vi "Add RPC Memeber VIs.vi"(8 "error in":errorcluster, 9 "Member VI Template Path":path=path "C:/dev/github/codegen/grpc-labview/labview source/Client Server Support New/gRPC Scripting Tools/Class API/MemberTemplate.vi", 10 "LVClassLibrary in":refnum<vi>, 11 "RPC Method Parameters":T1[](array[typedef])) -> (0 "error out":errorcluster, 2 "dynamic member VIs":refnum<vi>[](array[refnum]), 3 "LVClassLibrary out":refnum<vi>)   [LabVIEW 2019, in "gRPC Template Creation Utility.lvlib"]
uses:
  gRPC Template Creation Utility.lvlib
  TypeDefs/RPC Method Parameters.ctl
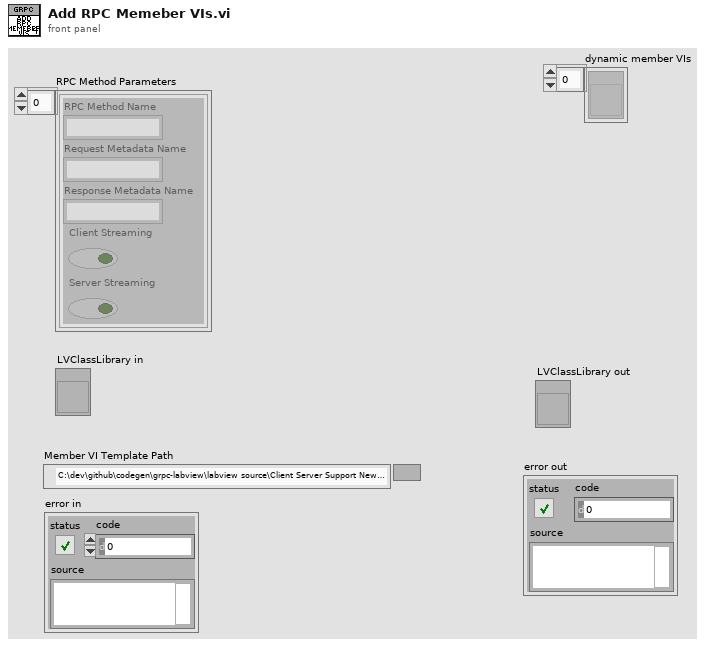
[diagram p1: front panel]
types:
  T1 = typedef "gRPC Template Creation Utility.lvlib/RPC Method Parameters.ctl" = cluster{"RPC Method Name":string, "Request Metadata Name":string, "Response Metadata Name":string, "Client Streaming":bool, "Server Streaming":bool}
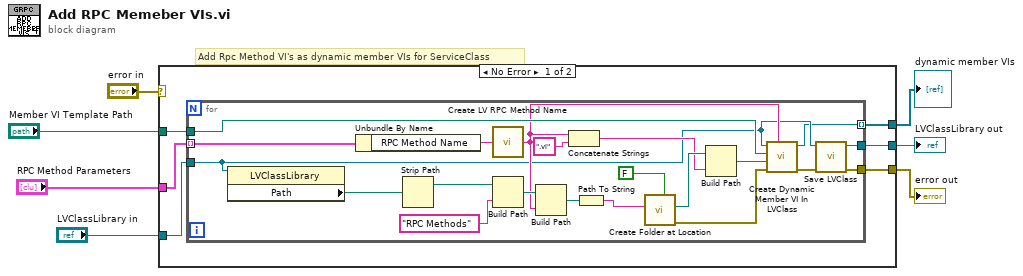
[diagram p0: block diagram]
diagram:
  # "Add Rpc Method VI's as dynamic member VIs for ServiceClass"
  n1 = case shown="No Error" "error in" {
    selector: "error in" -> [_ w36]
    tunnel: "RPC Method Parameters" -> [w13 _]
    tunnel: "LVClassLibrary in" -> [w12 w35]
    tunnel: [w11 w35] -> w4
    tunnel: "Member VI Template Path" -> [w10 _]
    tunnel: [w9 w36] -> w2
    tunnel: [w8 _] -> w1
    frame No Error {
      n2 = for {
        tunnel: w13 -> [w34] mode=indexing
        tunnel: w12 -> [w19]
        tunnel: [w15] -> w11
        tunnel: w10 -> [w30]
        tunnel: [w17] -> w9
        tunnel: [w14] -> w8 mode=indexing
        n3 = property class="LVClassLibrary"(reference=w19) -> ("Path"=w29:path)  [unwired: 1 in, 2 out]
        n4 = Unbundle By Name(w34) -> ("RPC Method Name"=w33:string)
        n5 = Strip Path(path=w29) -> (stripped path=w28:path)  [unwired: 1 out]
        n6 = call "Create LV RPC Method Name.vi"("Proto Parser RPC Method Name in"=w33) -> ("LV RPC Method Name out"=w20:string)
        n7 = Build Path(base path=w28, name or relative path="RPC Methods" ("Item Name")) -> (appended path=w26:path)
        n8 = Build Path(base path=w26, name or relative path=w20) -> (appended path=w24:path)
        n9 = Concatenate Strings(w20, ".vi" ("string")) -> (w21:string)
        n10 = Path To String(path=w24) -> (string=w23:string)
        n11 = call "Create Folder at Location.vi"("Override existing (F)"=FALSE, "Path"=w23) -> ("Error Out"=w16:errorcluster, "Full path out"=w22:path)  [unwired: 7 in, 1 out]
        n12 = Build Path(base path=w22, name or relative path=w21) -> (appended path=w31:path)
        n13 = call "Create Dynamic Member VI In LVClass.vi"("RPC Method Name"=w20, "error in (no error)"=w16, "New VI Path"=w31, "Member VI Template Path"=w30, "LVClassLibrary in"=w19) -> ("error out"=w18:errorcluster, "dynamic member vi out"=w14:refnum<vi>)  [unwired: 5 in]
        n14 = call "Save LVClass.vi"("error in (no error)"=w18, "LVClassLibrary in"=w19) -> ("error out"=w17:errorcluster, "LVClassLibrary out"=w15:refnum<vi>)  [unwired: 8 in]
      }
    }
    frame Error {
    }
  }
  "LVClassLibrary out" <- w4
  "error out" <- w2
  "dynamic member VIs" <- w1
